vi "Add Files to Archive.vi"(8 "error in (no error)":errorcluster, 9 "relative paths in zip":path[](array[path]), 10 "absolute source paths":path[](array[path]), 11 "zip path":path) -> (0 "error out":errorcluster)   [LabVIEW 2020]
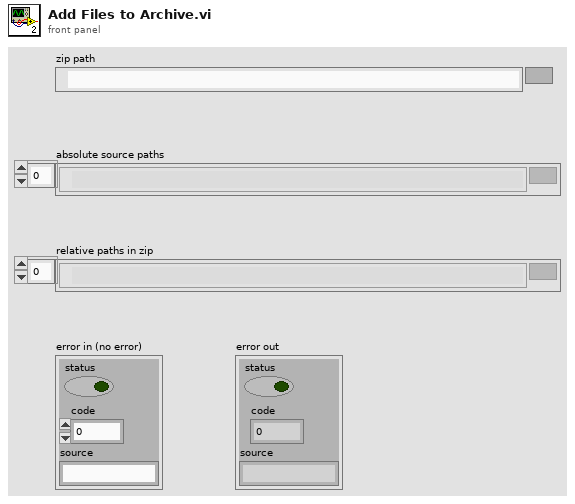
[diagram p1: front panel]
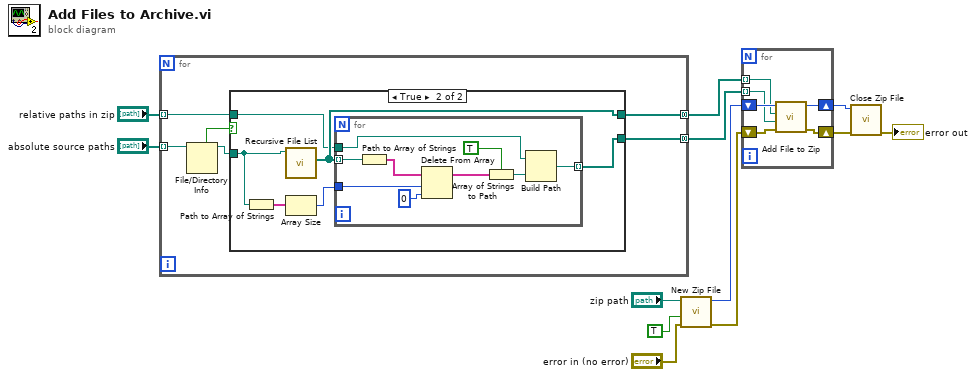
[diagram p0: block diagram]
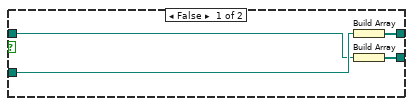
[diagram p2: hidden frame]
diagram:
  n1 = for {
    tunnel: [w16] -> w2 mode=concatenating
    tunnel: "absolute source paths" -> [w15] mode=indexing
    tunnel: "relative paths in zip" -> [w14] mode=indexing
    tunnel: [w13] -> w1 mode=concatenating
    n2 = File/Directory Info(path=w15) -> (path out=w17:path, directory=w18:bool)  [unwired: 1 in, 5 out]
    n3 = case shown="True" w18 {
      tunnel: w17 -> [w22 w24]
      tunnel: [w21 w28] -> w16
      tunnel: w14 -> [w20 w23]
      tunnel: [w19 w27] -> w13
      frame False {
        n4 = Build Array(w22) -> (w21:path[])
        n5 = Build Array(w20) -> (w19:path[])
      }
      frame True {
        n6 = Path to Array of Strings(0:w24) -> (2:w26:string[])  [unwired: 1 out]
        n7 = call <vilib>:"Recursive File List.vi"("Folder Path"=w24) -> ("All Files in Dir"=w28:path[])  [unwired: 6 in, 4 out]
        n8 = Array Size(array=w26) -> (size(s)=w25:i32)
        n9 = for {
          tunnel: w28 -> [w37] mode=indexing
          tunnel: [w35] -> w27 mode=indexing
          tunnel: w25 -> [w36]
          tunnel: w23 -> [w29]
          n10 = Path to Array of Strings(0:w37) -> (2:w33:string[])  [unwired: 1 out]
          n11 = Delete From Array(array=w33, length=w36, index=0 ("length")) -> (array with subset deleted=w31:string[])  [unwired: 1 out]
          n12 = Array of Strings to Path(0:w31, 1:TRUE ("relative")) -> (2:w30:path)
          n13 = Build Path(base path=w29, name or relative path=w30) -> (appended path=w35:path)
        }
      }
    }
  }
  n14 = call <vilib>:"New Zip File.vi"("error in (no error)"="error in (no error)", "confirm overwrite? (F)"=TRUE, "target"="zip path") -> ("error out"=w10:errorcluster, "zip file out"=w5:i64)  [unwired: 2 in, 1 out]
  n15 = for {
    tunnel: w2 -> [w38] mode=indexing
    shift-right: [w39] -> w9
    shift-left: w10 -> [w41]
    shift-right: [w42] -> w8
    shift-left: w5 -> [w43]
    tunnel: w1 -> [w40] mode=indexing
    n16 = call <vilib>:"Add File to Zip.vi"("error in (no error)"=w41, "destination path in zip"=w40, "source file path"=w38, "zip file in"=w43) -> ("error out"=w39:errorcluster, "zip file out"=w42:i64)  [unwired: 6 in]
  }
  n17 = call <vilib>:"Close Zip File.vi"("error in (no error)"=w9, "zip file in"=w8) -> ("error out"=→"error out":errorcluster)  [unwired: 5 in]
